vi "AuMT8852B EUT Address.vi"(5 "EUT Address (0x000000000000)":string="0x000000000000", 7 "Set/Get (Set)":enum16{"Set", "Get"}(ring), 8 "error in (no error)":errorcluster, 11 "VISA session":refnum<visa-resource-name>) -> (0 "error out":errorcluster, 2 "error code":i32, 3 "VISA session out":refnum<visa-resource-name>, 4 "EUT Address out":string)   [LabVIEW 2017]
doc: "Anritsu MT8852B Bluetooth Tester\n\nSets or retrieves the Bluetooth address of the EUT.\n\nINPUTS\nSet/Get - whether the value is being sent to or retrieved from the instrument.\nEUT Address - the address of the EUT\n\nOUTPUTS\nAddress out - the current EUT address."
uses:
  <instrlib>/aumt8852B/General/Utilities/MT8850 Attribute ID.ctl
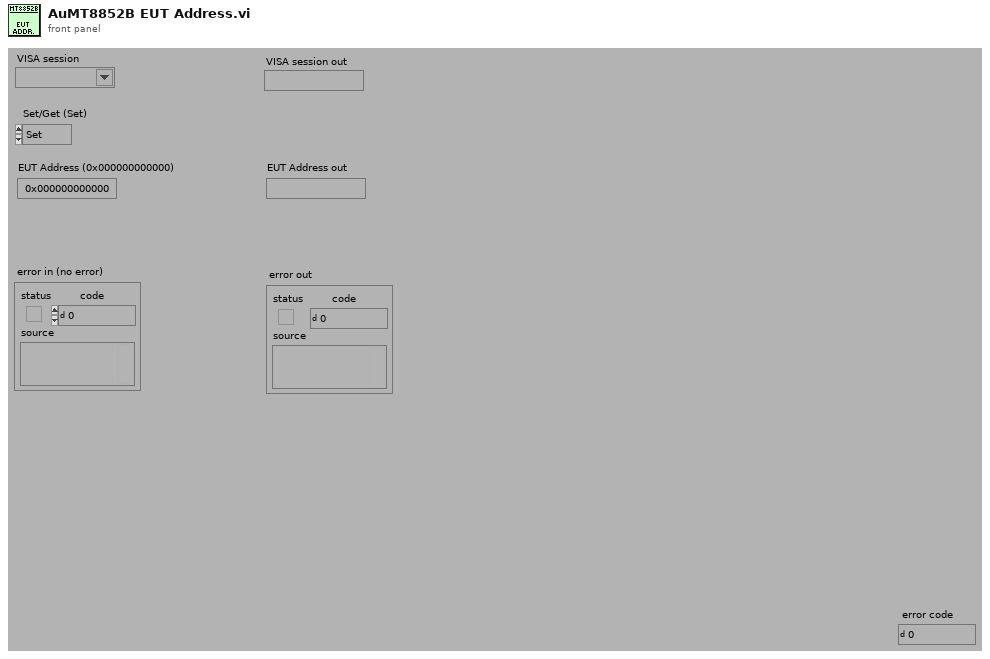
[diagram p1: front panel]
types:
  T1 = typedef "MT8850 Attribute ID.ctl" = enum16{"Operation mode", "Selected script", "EUT address source", "EUT Address", "EUT HCI RS232 Baud Rate", "Tester GPIB Address", "Tester RS232 Baud Rate", "Tester Bluetooth Address", "Tester Contrast", "Tester Key Click On", "Tester Modulation Index", "Tester Poll-Null Mode", "Tester Power Range", "Tester RS232 Mode", "Beep on Illegal Entry", "Display User Text", "User Text", "Calibration TX Modulation DAC", "Calibration RX Channel", "Calibration TX Channel", "Calibration TX Power", "Calibration Use TX Table", "Inquiry Request User-friendly Name", "Inquiry Number of Responses", "Inquiry Timeout", "Script Frequency Display", "Script Loop Count", "Script Loop Continuously", "Script Loop Stop on Fail", "Link timeout", "Page timeout", "Filter bandwidth", "SCO air code", "SCO bit position", "SCO input code", "SCO input data", "SCO input sample size", "SCO loopback mode", "SCO packet type", "SCO tone generator", "Tester page scan repetition mode", "Tester follow test mode", "Tester authentication state", "Tester authentication pin code", "Tester authentication pin length"}
  T2 = typedef "Attribute Status.ctl" = enum16{"No I/O needed", "I/O needed"}
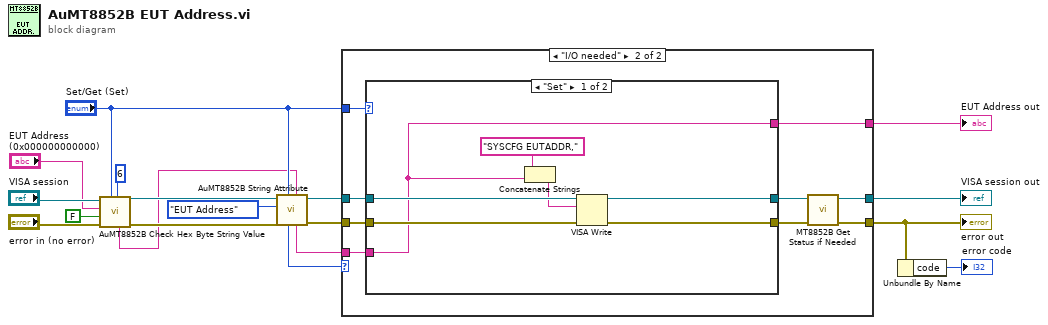
[diagram p0: block diagram]
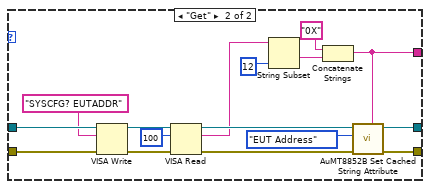
[diagram p3: hidden frame]
diagram:
  n1 = call <instrlib>:"AuMT8852B Check Hex Byte String Value.vi"("Number of bytes (6)"=6, "Set/Get (Set)"="Set/Get (Set)", "error in (no error)"="error in (no error)", "Check IVI flag first? (T)"=FALSE, "Hex byte string (0)"="EUT Address (0x000000000000)", "VISA session"="VISA session") -> ("error out"=w10:errorcluster, "VISA session out"=w11:refnum<visa-resource-name>, "Hex byte string out"=w4:string)  [unwired: 3 in]
  n2 = call <instrlib>:"AuMT8852B String Attribute.vi"("Value (\"\")"=w4, "Set/Get (Set)"="Set/Get (Set)", "error in (no error)"=w10, "Attribute ID"=MT8850_Attribute_ID."EUT Address", "VISA session"=w11) -> ("error out"=w14:errorcluster, "VISA session out"=w15:refnum<visa-resource-name>, "Value out"=w17:string, "Status"=w13:T2)  [unwired: 3 in]
  n3 = case shown="\"I/O needed\"" w13 {
    tunnel: "Set/Get (Set)" -> [_ w30]
    tunnel: w17 -> [w21 w29]
    tunnel: [w19 w22] -> w2
    tunnel: [w20 w23] -> w16
    tunnel: w15 -> [w20 w28]
    tunnel: w14 -> [w19 w27]
    tunnel: [w21 w26] -> w12
    frame "No I/O needed", Default {
    }
    frame "I/O needed" {
      n4 = case shown="\"Set\"" w30 {
        tunnel: [w34 w44] -> w24
        tunnel: w29 -> [w31 _]
        tunnel: [w35 w45] -> w25
        tunnel: w28 -> [w37 w53]
        tunnel: w27 -> [w36 w52]
        tunnel: [w31 w40] -> w26
        frame "Set" {
          n5 = Concatenate Strings("SYSCFG EUTADDR," ("Format String"), w31) -> (w32:string)
          n6 = VISA Write(VISA resource name=w37, write buffer=w32, error in (no error)=w36) -> (VISA resource name out=w35:refnum<visa-resource-name>, error out=w34:errorcluster)  [unwired: 1 out]
        }
        frame "Get" {
          n7 = VISA Write(VISA resource name=w53, write buffer="SYSCFG? EUTADDR" ("write buffer (\"\")"), error in (no error)=w52) -> (VISA resource name out=w51:refnum<visa-resource-name>, error out=w48:errorcluster)  [unwired: 1 out]
          n8 = VISA Read(VISA resource name=w51, byte count=u32 100 ("byte count (0)"), error in (no error)=w48) -> (VISA resource name out=w47:refnum<visa-resource-name>, read buffer=w42:string, error out=w46:errorcluster)  [unwired: 1 out]
          n9 = String Subset(string=w42, length (rest)=12) -> (substring=w39:string)  [unwired: 1 in]
          n10 = Concatenate Strings("0X", w39) -> (w40:string)
          n11 = call <instrlib>:"AuMT8852B Set Cached String Attribute.vi"("Value (\"\")"=w40, "error in (no error)"=w46, "Attribute ID"=MT8850_Attribute_ID."EUT Address", "VISA session"=w47) -> ("error out"=w44:errorcluster, "VISA session out"=w45:refnum<visa-resource-name>)  [unwired: 6 in]
        }
      }
      n12 = call <instrlib>:"MT8852B Get Status if Needed.vi"("error in (no error)"=w24, "VISA session"=w25) -> ("error out"=w22:errorcluster, "VISA session out"=w23:refnum<visa-resource-name>)  [unwired: 8 in]
    }
  }
  "error out" <- w2
  "VISA session out" <- w16
  "EUT Address out" <- w12
  n13 = Unbundle By Name(w2) -> ("code"=→"error code":i32)
